vi "libssh2_channel_forward_listen_ex - invalid session - no error 1097.vi"() -> ()   [LabVIEW 2013, in "libssh2_tests.lvlib"]
uses:
  libssh2_tests.lvlib
  libssh2/Session Refnum.ctl
  libssh2/libssh2_init_default.vi
  <vilib>/Utility/error.llb/General Error Handler.vi
  <vilib>/addons/_JKI Toolkits/Caraya/classes/Assert/Assert.vi
  <vilib>/addons/_JKI Toolkits/Caraya/classes/Assert/Assert Not Error.vi
  libssh2/libssh2.lvlib
  <vilib>/addons/_JKI Toolkits/Caraya/classes/Test/Test.lvclass
panel:
  out "error out":errorcluster
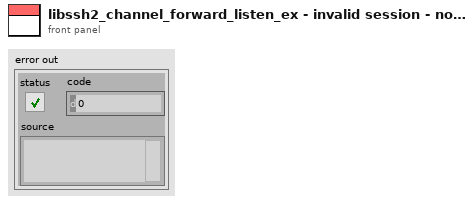
[diagram p1: front panel]
types:
  T1 = typedef "libssh2.lvlib/Session Refnum.ctl" = refnum<k1>
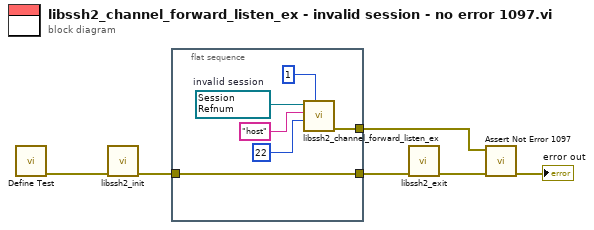
[diagram p0: block diagram]
diagram:
  n1 = call <vilib>:"Define Test.vi"() -> ("error out"=w6:errorcluster)  [unwired: 10 in, 1 out]
  n2 = call-poly "libssh2_init.vi"("error in (no error)"=w6) -> ("error out"=w4:errorcluster)  [unwired: 10 in]
  n3 = flat-sequence {
    tunnel: [w12] -> w3
    tunnel: w4 -> [w12]
    tunnel: [w11] -> w2
    frame #0 {
      w10 = T1 refnum items=["Session"]  # invalid session
      n4 = call "libssh2_channel_forward_listen_ex.vi"("queue_maxsize"=1, "port"=22, "host"="host", "session"=w10) -> ("error out"=w11:errorcluster)  [unwired: 5 in, 2 out]
    }
  }
  n5 = call "libssh2_exit.vi"("error in (no error)"=w3) -> ("error out"=w5:errorcluster)  [unwired: 10 in]
  n6 = call "Assert Not Error 1097.vi"("error in (no error)"=w5, "actual value"=w2) -> ("error out"=→"error out":errorcluster)  [unwired: 9 in]
